vi "power_supply.vi"() -> ()   [LabVIEW 2014]
panel:
  out "读取缓冲区":string
  in  "错误输入（无错误）":errorcluster
  out "错误输出":errorcluster
  in  "commend":string
  in  "地址输入":string
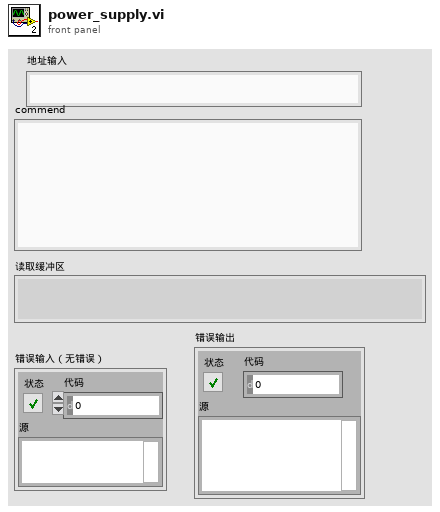
[diagram p1: front panel]
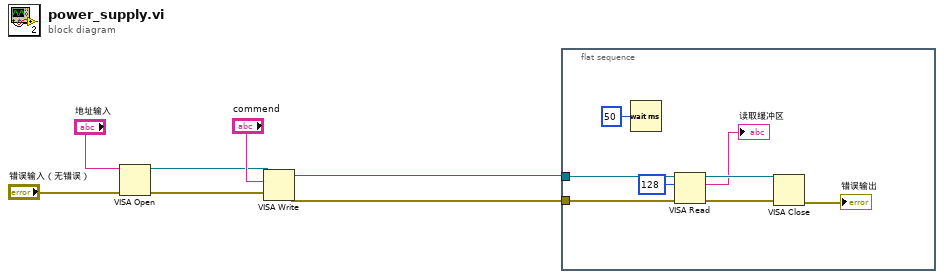
[diagram p0: block diagram]
diagram:
  n1 = VISA Open(error in (no error)="错误输入（无错误）", VISA resource name="地址输入") -> (VISA resource name=w6:refnum<visa-resource-name>, error out=w5:errorcluster)  [unwired: 3 in]
  n2 = VISA Write(VISA resource name=w6, write buffer="commend", error in (no error)=w5) -> (VISA resource name out=w2:refnum<visa-resource-name>, error out=w1:errorcluster)  [unwired: 1 out]
  n3 = flat-sequence {
    tunnel: w2 -> [w12]
    tunnel: w1 -> [w9]
    frame #0 {
      n4 = Wait (ms)(milliseconds to wait=u32 50 ("等待时间（毫秒）")) -> ()  [unwired: 1 out]
      n5 = VISA Read(VISA resource name=w12, byte count=u32 128 ("字节总数"), error in (no error)=w9) -> (VISA resource name out=w14:refnum<visa-resource-name>, read buffer=→"读取缓冲区":string, error out=w13:errorcluster)  [unwired: 1 out]
      n6 = VISA Close(VISA resource name=w14, error in (no error)=w13) -> (error out=→"错误输出":errorcluster)
    }
  }
